vi "CRYCustom Step Function.vi"(6 "bData":bool, 7 "sAction":string, 8 "VI Ref":refnum<vi>, 10 "sData":string, 11 "nData":i32) -> (0 "bData Out":bool, 2 "sData Out":string)   [LabVIEW 2013]
uses:
  CRYStepSetup/CRYStepSetup Global.vi
  CRYMainGlobal.vi
  Program/CRYRef nums global.vi
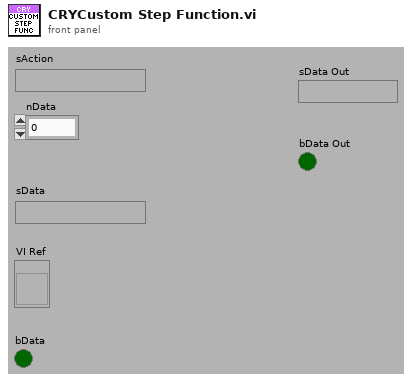
[diagram p1: front panel]
types:
  T1 = enum16{"open", "replace", "create", "open or create", "replace or create", "replace or create with confirmation"}
  T2 = typedef "CRYStep.ctl" = cluster{"No.VI":i32, "Category":string, "StepName":string, "Seq setup flattened":string, "Comment":string, "Steps config.":bool[], "Jump config":i32[], "Start":dbl, "Increment":dbl, "Name":string, "Unit":string, "Y data":u16, "Y prefix":string, "Y dB ref":dbl, "Y unit":string, "Repeat State Array":cluster{"Start":dbl, "Increment":dbl, "Count":i32, "Num":i32}[]}
  T3 = typedef "CRYCustom Cluster.ctl" = cluster{"Help":string, "Flatten Data":string}
  T4 = enum16{"big-endian, network order", "native, host order", "little-endian"}
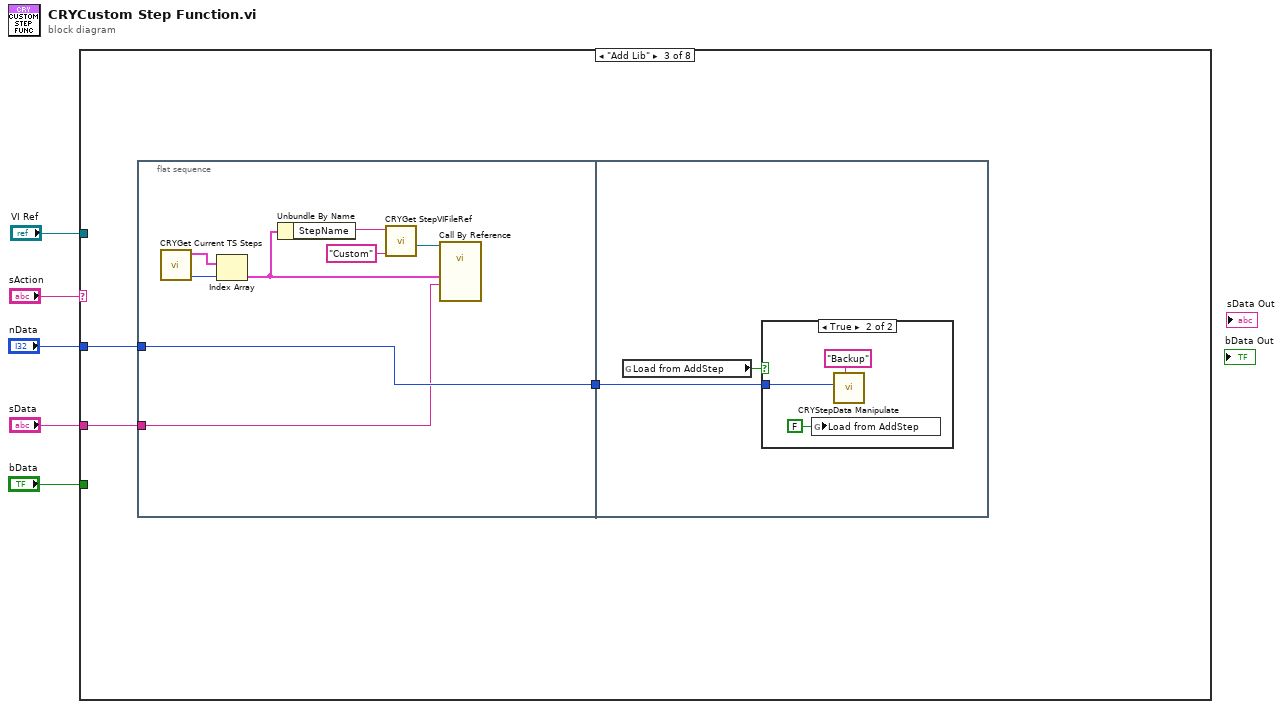
[diagram p0: block diagram]
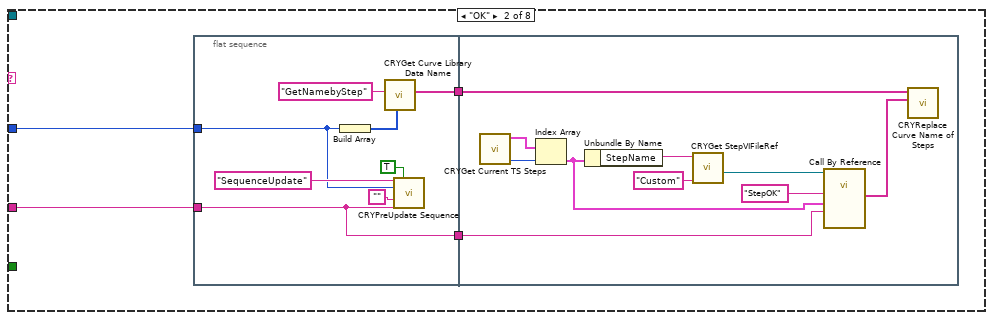
[diagram p3: hidden frame]
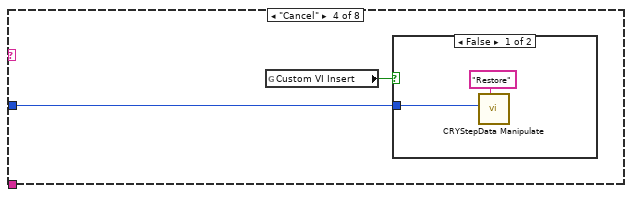
[diagram p5: hidden frame]
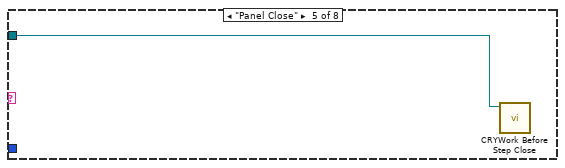
[diagram p7: hidden frame]
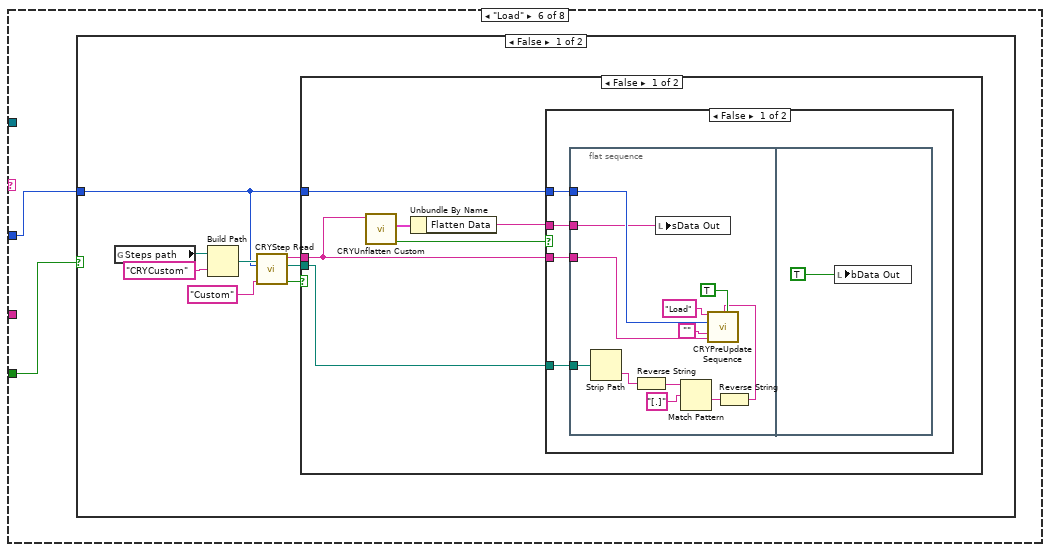
[diagram p8: hidden frame]
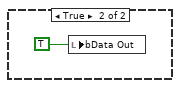
[diagram p11: hidden frame]
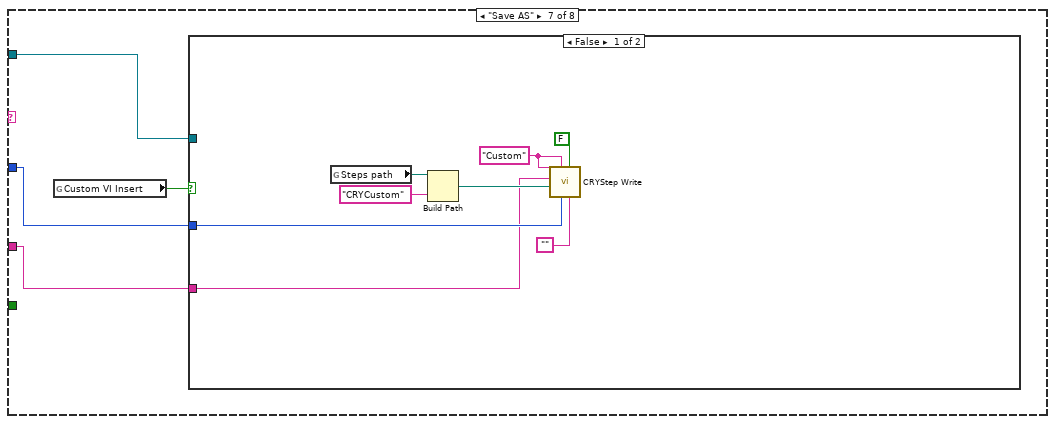
[diagram p12: hidden frame]
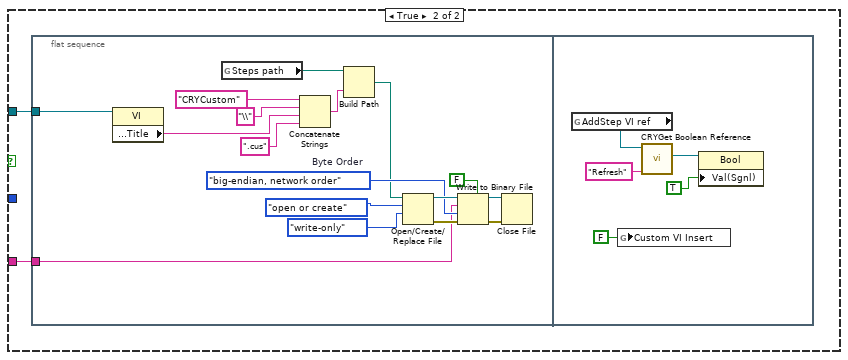
[diagram p13: hidden frame]
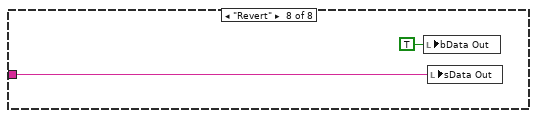
[diagram p14: hidden frame]
diagram:
  n1 = case shown="\"Add Lib\"" "sAction" {
    tunnel: "nData" -> [_ w7 w29 w44 _ w50 w83 _]
    tunnel: "sData" -> [_ w6 w28 _ _ _ w84 w120]
    tunnel: "VI Ref" -> [_ _ _ _ w48 _ w85 _]
    tunnel: "bData" -> [_ _ _ _ _ w49 _ _]
    frame Default {
    }
    frame "OK" {
      n2 = flat-sequence {
        tunnel: w7 -> [w12]
        tunnel: w6 -> [w10]
        tunnel: [w11] -> w9
        tunnel: [w10] -> w8
        tunnel: w9 -> [w25]
        tunnel: w8 -> [w19]
        frame #0 {
          n3 = Build Array(w12) -> (w14:i32[])
          n4 = call "CRYGet Curve Library Data Name.vi"("nData"=w14, "sAction"="GetNamebyStep" ("sOption")) -> ("sNames"=w11:string[])  [unwired: 6 in, 3 out]
          n5 = call "CRYPreUpdate Sequence.vi"("EventName"="SequenceUpdate", "Proper VI No"=w12, "Project View Step Name Identifier Arg1"="", "Step flattened Arg2"=w10, "AllChangeFlg"=TRUE ("Name/Identifier")) -> ()  [unwired: 11 in]
        }
        frame #1 {
          n6 = call "CRYGet Current TS Steps.vi"() -> ("SelectStepNumber in Tree"=w27:i32, "Steps"=w26:T2[])  [unwired: 7 in, 3 out]
          n7 = Index Array(array=w26, index=w27) -> (element=w21:T2)
          n8 = Unbundle By Name(w21) -> ("StepName"=w22:string)
          n9 = call "CRYGet StepVIFileRef.vi"("Category"="Custom", "Step Name"=w22) -> ("Step Name Replace VI ref"=w23:refnum<vi>)  [unwired: 6 in, 2 out]
          n10 = call-by-ref "?"(reference=w23, "Step Setup in"=w19, "Setup in"=w21, "Type In"="StepOK") -> ("Inserted Names Out"=w18:string[])  [unwired: 9 in, 2 out]
          n11 = call "CRYReplace Curve Name of Steps.vi"("New Name"=w18, "Old Name"=w25) -> ()  [unwired: 9 in, 1 out]
        }
      }
    }
    frame "Add Lib" {
      n12 = flat-sequence {
        tunnel: [w36] -> w30
        tunnel: w29 -> [w36]
        tunnel: w28 -> [w33]
        tunnel: w30 -> [w39]
        frame #0 {
          n13 = call "CRYGet Current TS Steps.vi"() -> ("SelectStepNumber in Tree"=w38:i32, "Steps"=w37:T2[])  [unwired: 7 in, 3 out]
          n14 = Index Array(array=w37, index=w38) -> (element=w32:T2)
          n15 = Unbundle By Name(w32) -> ("StepName"=w31:string)
          n16 = call "CRYGet StepVIFileRef.vi"("Category"="Custom", "Step Name"=w31) -> ("Step Name Replace VI ref"=w34:refnum<vi>)  [unwired: 6 in, 2 out]
          n17 = call-by-ref "?"(reference=w34, "Step Setup in"=w33, "Setup in"=w32) -> ()  [unwired: 10 in, 3 out]
        }
        frame #1 {
          n18 = global read "CRYStepSetup Global.vi" "Load from AddStep"() -> (w40:bool)
          n19 = case shown="True" w40 {
            tunnel: w39 -> [_ w42]
            frame False {
            }
            frame True {
              n20 = global write "CRYStepSetup Global.vi" "Load from AddStep"(FALSE ("Load from AddStep")) -> ()
              n21 = call "CRYStepData Manipulate.vi"("sAction"="Backup", "StepNo."=w42) -> ()  [unwired: 10 in]
            }
          }
        }
      }
    }
    frame "Cancel" {
      n22 = global read "CRYStepSetup Global.vi" "Custom VI Insert"() -> (w45:bool)
      n23 = case shown="False" w45 {
        tunnel: w44 -> [w46 _]
        frame False {
          n24 = call "CRYStepData Manipulate.vi"("sAction"="Restore", "StepNo."=w46) -> ()  [unwired: 10 in]
        }
        frame True {
        }
      }
    }
    frame "Panel Close" {
      n25 = call "CRYWork Before Step Close.vi"("StepVI Ref"=w48) -> ()  [unwired: 11 in]
    }
    frame "Load" {
      n26 = case shown="False" w49 {
        tunnel: w50 -> [w51 _]
        frame False {
          n27 = global read "CRYMainGlobal.vi" "Steps path"() -> (w57:path)
          n28 = Build Path(base path=w57, name or relative path="CRYCustom") -> (appended path=w58:path)
          n29 = call "CRYStep Read.vi"("Category Name"="Custom" ("Step File Name"), "Proper VI No"=w51, "Step File Path"=w58) -> ("status"=w52:bool, "selected path"=w53:path, "Flatten Step"=w54:string)  [unwired: 1 in, 3 out]
          n30 = case shown="False" w52 {
            tunnel: w51 -> [w64 _]
            tunnel: w54 -> [w61 _]
            tunnel: w53 -> [w63 _]
            frame False {
              n31 = call "CRYUnflatten Custom.vi"("Unflatten Custom"=w61) -> ("Error?"=w60:bool, "Custom"=w62:T3)  [unwired: 8 in, 1 out]
              n32 = Unbundle By Name(w62) -> ("Flatten Data"=w59:string)
              n33 = case shown="False" w60 {
                tunnel: w64 -> [w65 _]
                tunnel: w59 -> [w66 _]
                tunnel: w61 -> [w68 _]
                tunnel: w63 -> [w67 _]
                frame False {
                  n34 = flat-sequence {
                    tunnel: w68 -> [w77]
                    tunnel: w67 -> [w76]
                    tunnel: w66 -> [w69]
                    tunnel: w65 -> [w75]
                    frame #0 {
                      n35 = Strip Path(path=w76) -> (name=w71:string)  [unwired: 1 out]
                      n36 = Reverse String(1:w71) -> (0:w73:string)
                      n37 = local write "sData Out"(w69) -> ()
                      n38 = Match Pattern(string=w73, regular expression="[.]") -> (after substring=w74:string)  [unwired: 4 out]
                      n39 = Reverse String(1:w74) -> (0:w70:string)
                      n40 = call "CRYPreUpdate Sequence.vi"("EventName"="Load", "StepName Arg3"=w70, "Proper VI No"=w75, "Project View Step Name Identifier Arg1"="", "Step flattened Arg2"=w77, "AllChangeFlg"=TRUE ("Name/Identifier")) -> ()  [unwired: 10 in]
                    }
                    frame #1 {
                      n41 = local write "bData Out"(TRUE ("Load Test")) -> ()
                    }
                  }
                }
                frame True {
                }
              }
            }
            frame True {
            }
          }
        }
        frame True {
          n42 = local write "bData Out"(TRUE ("Load Test Out")) -> ()
        }
      }
    }
    frame "Save AS" {
      n43 = global read "CRYStepSetup Global.vi" "Custom VI Insert"() -> (w86:bool)
      n44 = case shown="False" w86 {
        tunnel: w83 -> [w88 _]
        tunnel: w84 -> [w87 w96]
        tunnel: w85 -> [_ w95]
        frame False {
          w94 = "Custom" ("Step File Name")
          n45 = global read "CRYMainGlobal.vi" "Steps path"() -> (w93:path)
          n46 = Build Path(base path=w93, name or relative path="CRYCustom") -> (appended path=w91:path)
          n47 = call "CRYStep Write.vi"("StepIdentifier"="", "Default"=FALSE, "Proper VI No"=w88, "Category Name"=w94, "Step File Path"=w91, "Step flattened"=w87, "Step File Name"=w94) -> ()  [unwired: 1 in, 4 out]
        }
        frame True {
          n48 = flat-sequence {
            tunnel: w96 -> [w98]
            tunnel: w95 -> [w97]
            frame #0 {
              w109 = T4."big-endian, network order"  # Byte Order
              n49 = property class="VI"(reference=w97) -> ("Front Panel.Title"=w101:string)  [unwired: 1 in, 2 out]
              n50 = global read "CRYMainGlobal.vi" "Steps path"() -> (w113:path)
              n51 = Concatenate Strings("CRYCustom", "\\" ("string"), w101, ".cus" ("string")) -> (w99:string)
              n52 = Build Path(base path=w113, name or relative path=w99) -> (appended path=w104:path)
              n53 = Open/Create/Replace File(file path (use dialog)=w104, operation (0:open)=T1."open or create", access (0:read/write)=enum16{"read/write", "read-only", "write-only"}."write-only") -> (refnum out=w112:refnum<file>, error out=w106:errorcluster)  [unwired: 1 in, 3 out]
              n54 = Write to Binary File(file (use dialog)=w112, data=w98, error in=w106, 5:FALSE ("prepend array or string size? (T)"), 9:w109) -> (refnum out=w107:refnum<file>, error out=w105:errorcluster)  [unwired: 2 out]
              n55 = Close File(refnum=w107, error in=w105) -> ()  [unwired: 2 out]
            }
            frame #1 {
              n56 = global read "CRYRef nums global.vi" "AddStep VI ref"() -> (w115:refnum<vi>)
              n57 = global write "CRYStepSetup Global.vi" "Custom VI Insert"(FALSE ("Custom VI Insert")) -> ()
              n58 = call "CRYGet Boolean Reference.vi"("Label Name"="Refresh", "VI Refnum"=w115) -> ("Boolean Ref"=w117:refnum<vi>)  [unwired: 7 in, 2 out]
              n59 = property class="Bool"(reference=w117, "Val(Sgnl)"=TRUE ("element")) -> ()  [unwired: 1 in, 2 out]
            }
          }
        }
      }
    }
    frame "Revert" {
      n60 = local write "bData Out"(TRUE ("bData Out")) -> ()
      n61 = local write "sData Out"(w120) -> ()
    }
  }
